vi "CMD_VIDEO.vi"(6 "Gantry in":refnum<class "Gantry.lvclass">, 8 "error in (no error)":errorcluster, 10 "Arguments":string[](array[string]), 11 "gScript Interpreter in":refnum<class "gScript Interpreter.lvclass">) -> (0 "error out":errorcluster, 1 "Pause out":bool, 3 "gScript Interpreter out":refnum<class "gScript Interpreter.lvclass">, 4 "Gantry out":refnum<class "Gantry.lvclass">)   [LabVIEW 2024, in "gScript Interpreter.lvclass"]
uses:
  gScript Interpreter.lvclass
  Shared Components/Gantry Class/Gantry.lvclass
  Shared Components/Vec3d Class/Vec3d.lvclass
  Shared Components/Utils/Type Definitions/Physical Image.ctl
  <vilib>/vision/Image Controls.llb/IMAQ Image.ctl
  Shared Components/FlexWorktable/FlexWorktable.lvclass
  gScript Interpreter.lvclass/gScript Interpreter.ctl
  Shared Components/Vision/Vision.lvlib
panel:
  in  "Snapshot":bool
  in  "Point B Image":refnum<class "Vec3d.lvclass">
  in  "Point A Image":refnum<class "Vec3d.lvclass">
  in  "Point B":refnum<class "Vec3d.lvclass">
  in  "Point A":refnum<class "Vec3d.lvclass">
  in  "Mode Selection":enum32{"Motion", "Measure"}(radio)
  out "Error List":map{string, u64}(c390)
  out "FPS":string
  out "Reference Image":T1(plugin-control)
  in  "Autofocus":bool
  in  "Copy Button":bool
  in  "Pause on Exit":bool
  in  "Light Intensity":i32(slide) scale=0.0..100.0
  in  "Crosshair":bool
  out "Z":dbl format="%.3f"
  out "Y":dbl format="%.3f"
  out "X":dbl format="%.3f"
  in  "Continue":bool
  out "Preview":T1(plugin-control)
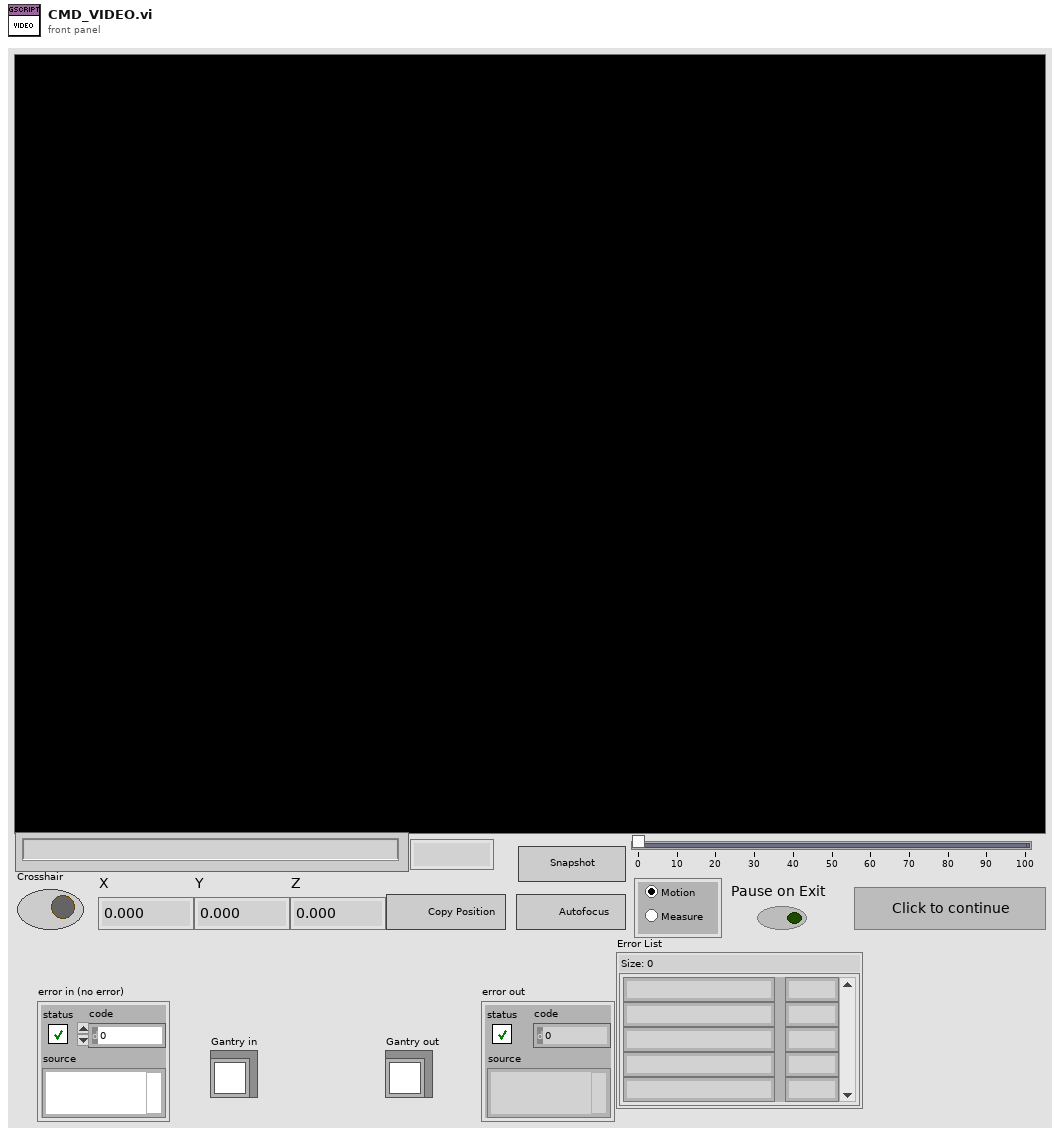
[diagram p1: front panel]
types:
  T1 = typedef "IMAQ Image.ctl" = refnum<image>
  T2 = typedef "Physical Image.ctl" = cluster{"Image Position":refnum<class "Vec3d.lvclass">, "Image Reference":T1, "Field of View":cluster{"x(mm)":dbl, "y(mm)":dbl}}
  T3 = cluster{"Left":i32, "Top":i32, "Right":i32, "Bottom":i32}
  T4 = typedef "FlexWorktable.lvclass/Camera State.ctl" = cluster{"Group":i32, "Open?":bool, "Driver":T5, "serial number":string, "Field of View":cluster{"x-mm":dbl, "y-mm":dbl}, "Rotation":T6, "Vertical Mirror":bool}
  T5 = typedef "Vision.lvlib/camera driver.ctl" = enum16{"none", "wmf", "imaqdx", "peak"}
  T6 = typedef "Camera Rotation.ctl" = enum16{"0", "90", "180", "270"}
  T7 = cluster{"Shift":bool, "Ctrl":bool, "Alt":bool, "Cmd":bool, "Opt":bool}
  T8 = typedef "Vision.lvlib/camera.ctl" = cluster{"camera reference":variant, "driver":T5, "identifier":string}
  T9 = typedef "LVPoint32TypeDef.ctl" = cluster{"Horizontal":i32, "Vertical":i32}
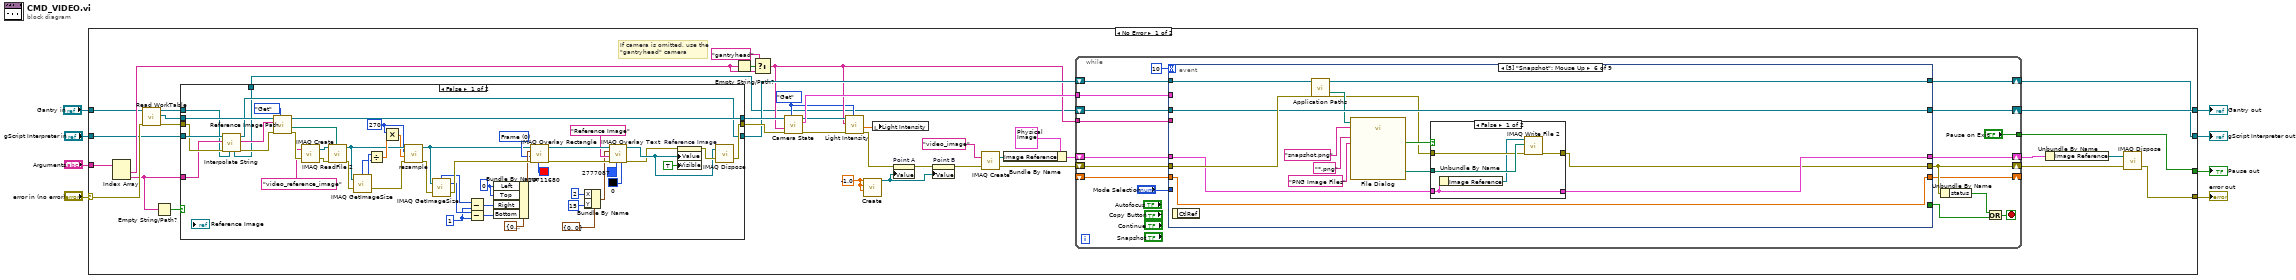
[diagram p0: block diagram]
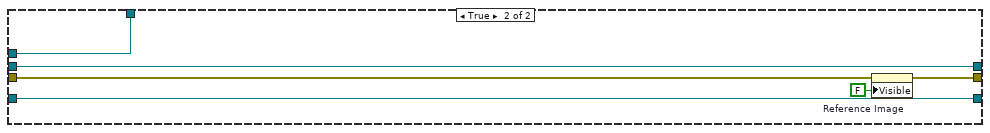
[diagram p2: hidden frame]
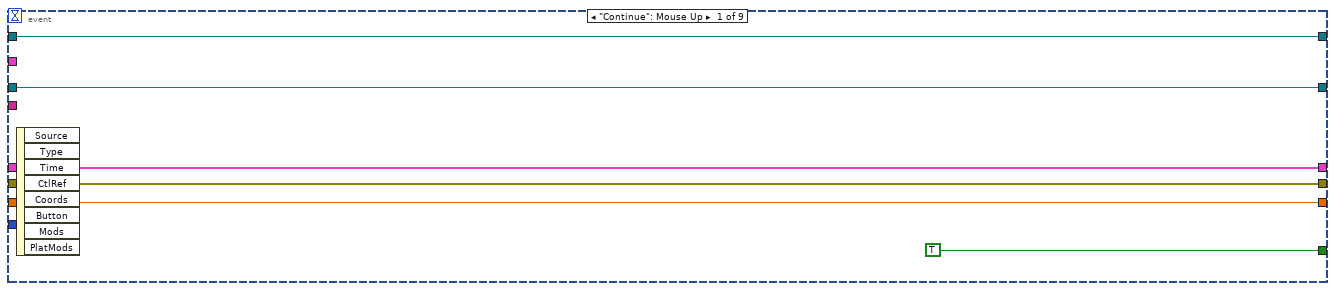
[diagram p3: hidden frame]
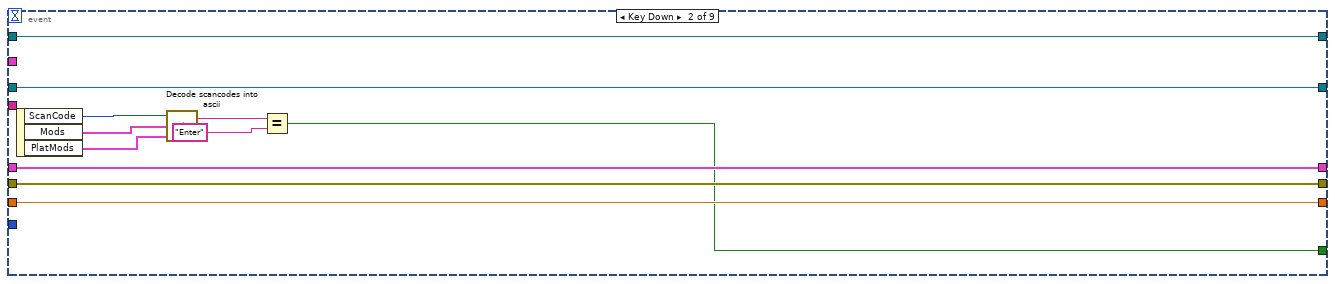
[diagram p4: hidden frame]
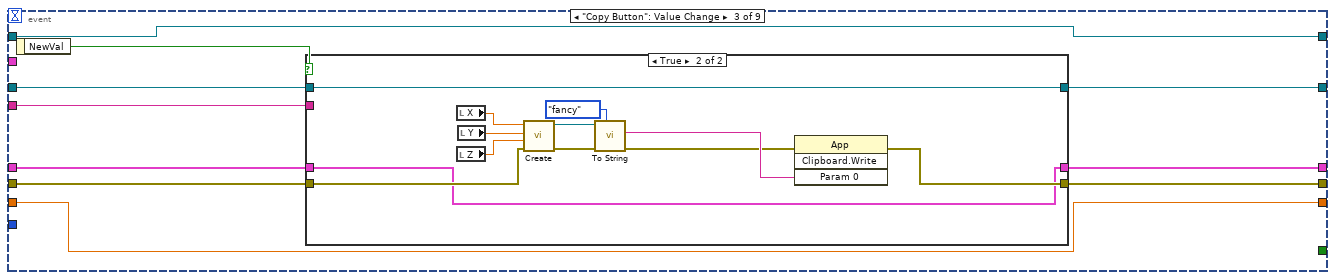
[diagram p5: hidden frame]
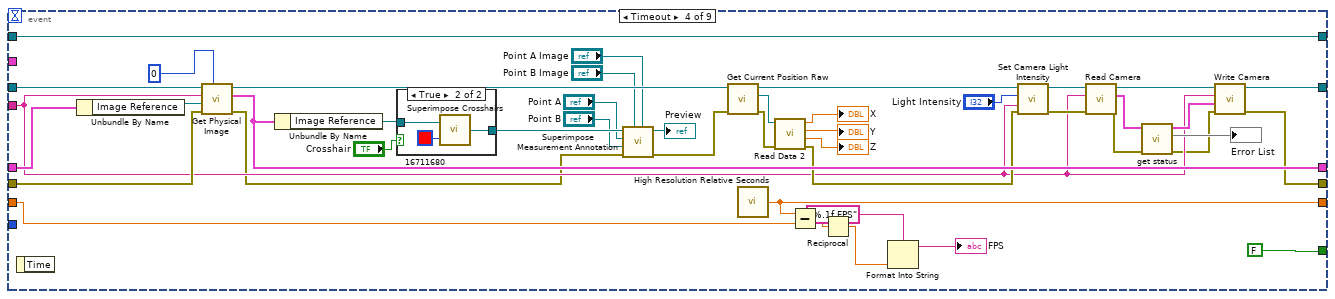
[diagram p7: hidden frame]
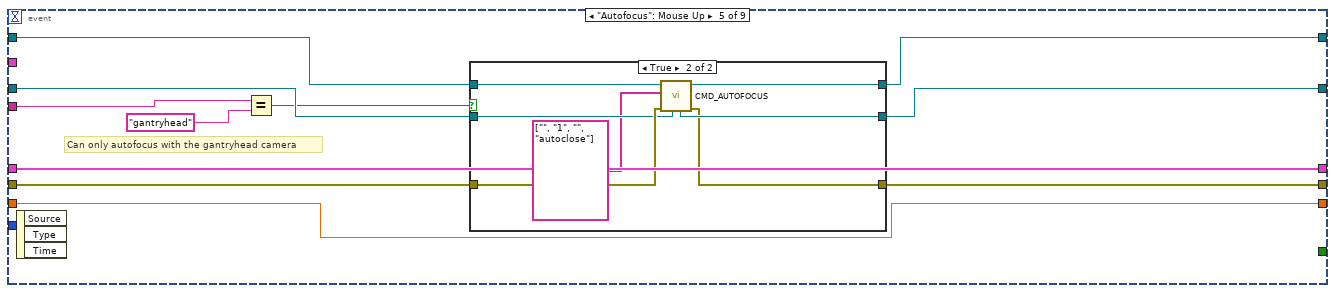
[diagram p9: hidden frame]
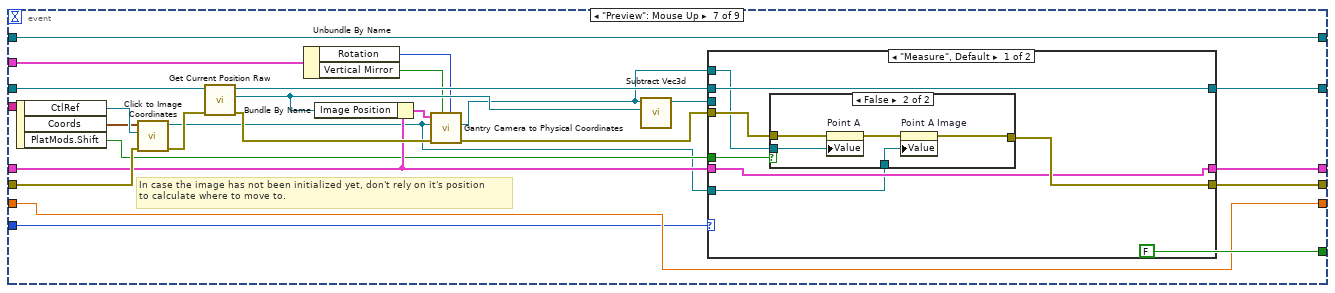
[diagram p12: hidden frame]
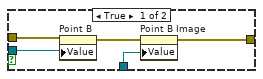
[diagram p13: hidden frame]
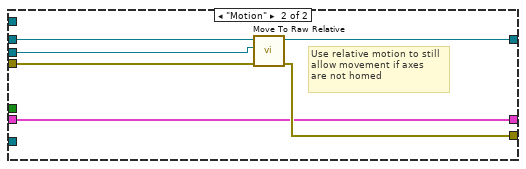
[diagram p14: hidden frame]
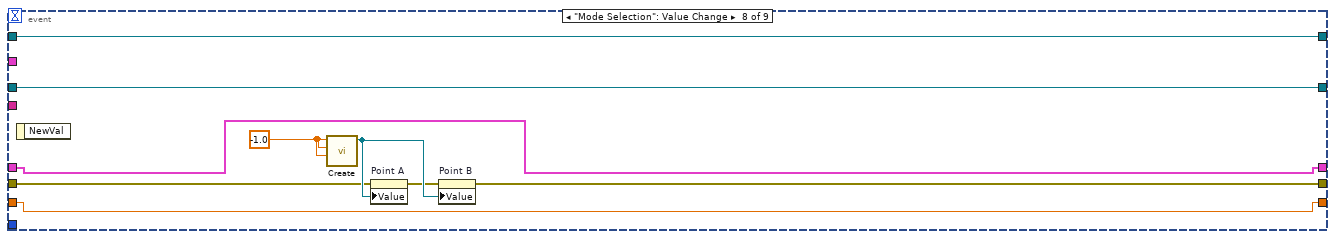
[diagram p15: hidden frame]
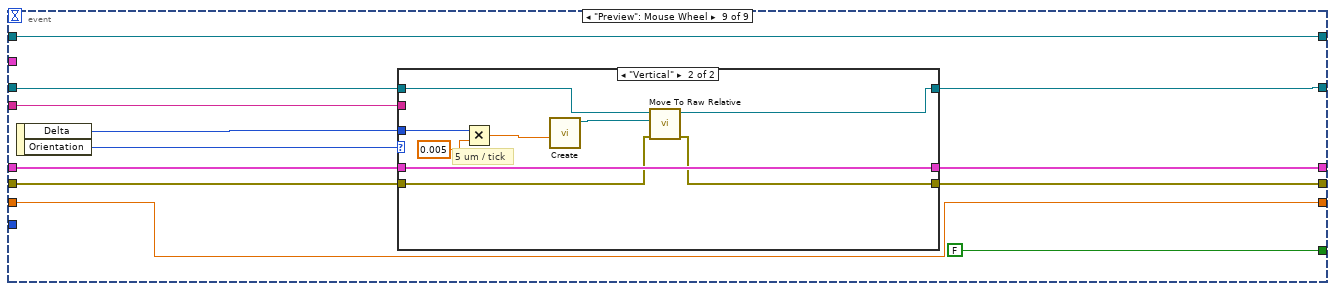
[diagram p16: hidden frame]
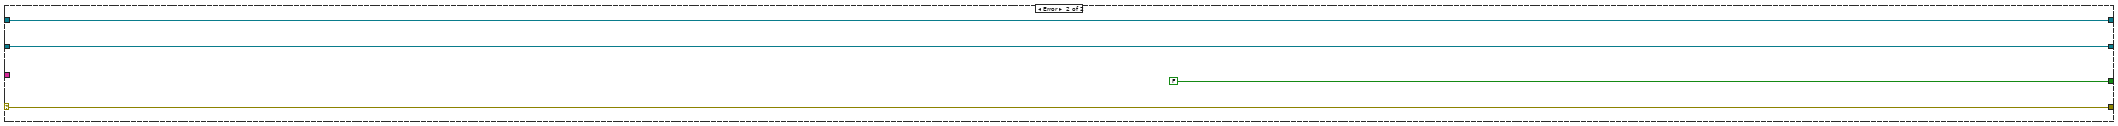
[diagram p18: hidden frame]
diagram:
  n1 = case shown="No Error" "error in (no error)" {
    selector: "error in (no error)" -> [w29 w340]
    tunnel: [w45 w340] -> w7
    tunnel: [w32 w339] -> w5
    tunnel: "gScript Interpreter in" -> [w22 w339]
    tunnel: "Arguments" -> [w47 _]
    tunnel: "Gantry in" -> [w31 w338]
    tunnel: [w46 w338] -> w2
    tunnel: [w33 FALSE ("Pause on Exit")] -> w1
    frame No Error {
      w12 = -1.0 ("X")
      w17 = enum16{"Get", "Set"}."Get" ("Get/Set")
      # "If camera is omitted, use the\n\"gantryhead\" camera"
      n2 = Index Array(array=w47) -> (element #1=w43:string, element #2=w26:string)  [unwired: 2 in]
      n3 = call-dynamic "Read WorkTable.vi"("error in"=w29, "Gantry Class in"=w31) -> ("error out"=w24:errorcluster, "Worktable"=w28:refnum<class "FlexWorktable.lvclass">, "Gantry Class out"=w10:refnum<class "Gantry.lvclass">)  [unwired: 7 in]
      n4 = Empty String/Path?(string/path=w26) -> (empty?=w27:bool)
      n5 = case shown="False" w27 {
        tunnel: w28 -> [w52 w104]
        tunnel: w26 -> [w54 _]
        tunnel: [w92 w104] -> w25
        tunnel: w24 -> [w55 w102]
        tunnel: [w90 w101] -> w23
        tunnel: w22 -> [w56 w100]
        tunnel: [w50 w100] -> w21
        tunnel: w10 -> [w49 w99]
        tunnel: [w48 w99] -> w9
        frame False {
          w58 = 270 ("X Resolution")
          w78 = u32 0 items=["Frame", "Fill", "Highlight"] ("Drawing Mode (Frame)")
          w80 = 1 ("y")
          w85 = 0 ("Left")
          n6 = call-dynamic "Interpolate String.vi"("Gantry in"=w49, "error in (no error)"=w55, "Input String"=w54, "gScript Interpreter in"=w56) -> ("error out"=w51:errorcluster, "Output String"=w53:string, "gScript Interpreter out"=w50:refnum<class "gScript Interpreter.lvclass">, "Gantry out"=w48:refnum<class "Gantry.lvclass">)  [unwired: 4 in]
          n7 = call "Reference Image Path.vi"("Get/Set"=enum16{"Get", "Set"}."Get", "error in (no error)"=w51, "Image ID/Path"=w53, "FlexWorktable in"=w52) -> ("error out"=w95:errorcluster, "Image Path"=w97:path, "FlexWorktable out"=w92:refnum<class "FlexWorktable.lvclass">)  [unwired: 5 in]
          n8 = call "IMAQ Create"("Image Name"="video_reference_image", "error in (no error)"=w95) -> ("New Image"=w96:T1, "error out"=w94:errorcluster)  [unwired: 3 in]
          n9 = call "IMAQ ReadFile 2"("File Path"=w97, "error in (no error)"=w94, "Image"=w96) -> ("error out"=w66:errorcluster, "Image Out"=w60:T1)  [unwired: 4 in, 3 out]
          n10 = call "IMAQ GetImageSize"("Image"=w60, "error in (no error)"=w66) -> ("Y Resolution"=w65:i32, "X Resolution"=w64:i32, "error out"=w61:errorcluster)  [unwired: 2 in]
          n11 = Divide(x=w65, y=w64) -> (x/y=w63:dbl)
          n12 = Multiply(x=w58, y=w63) -> (x*y=w57:dbl)
          n13 = call "resample.vi"("error in (no error)"=w61, "Height"=w57, "Width"=w58, "Image in"=w60) -> ("error out"=w62:errorcluster, "Image out"=w59:T1)  [unwired: 6 in]
          n14 = call "IMAQ GetImageSize"("Image"=w59, "error in (no error)"=w62) -> ("Y Resolution"=w81:i32, "X Resolution"=w82:i32, "error out"=w87:errorcluster)  [unwired: 2 in]
          n15 = Subtract(x=w82, y=w80) -> (x-y=w83:i32)
          n16 = Subtract(x=w81, y=w80) -> (x-y=w79:i32)
          n17 = Bundle By Name(cluster=T3 {"Left"=0, "Top"=0, "Right"=0, "Bottom"=0} ("Rectangle"), "Left"=w85, "Top"=w85, "Right"=w83, "Bottom"=w79) -> (w84:T3)
          n18 = call "IMAQ Overlay Rectangle"("Color"=u32 16711680, "error in (no error)"=w87, "Drawing Mode (Frame)"=w78, "Rectangle"=w84, "Image"=w59) -> ("error out"=w77:errorcluster, "Image Out"=w76:T1)  [unwired: 5 in]
          n19 = Bundle By Name(cluster=cluster{"X":i32, "Y":i32} {"X"=0, "Y"=0} ("Origin"), "X"=2, "Y"=15) -> (w69:cluster{"X":i32, "Y":i32})
          n20 = call "IMAQ Overlay Text"("BG Color (Transparent)"=u32 0, "Text Color (black)"=u32 2777087, "error in (no error)"=w77, "String"="Reference Image", "Origin"=w69, "Image"=w76) -> ("error out"=w74:errorcluster, "Image Out"=w75:T1)  [unwired: 4 in]
          n21 = property on="Reference Image" class="ImageControl"(error in=w74, "Value"=w75, "Visible"=TRUE) -> (error out=w91:errorcluster)  [unwired: 1 in, 1 out]
          n22 = call "IMAQ Dispose"("Image"=w75, "error in (no error)"=w91) -> ("error out"=w90:errorcluster)  [unwired: 4 in]
        }
        frame True {
          n23 = property on="Reference Image" class="ImageControl"(error in=w102, "Visible"=FALSE) -> (error out=w101:errorcluster)  [unwired: 1 in, 1 out]
        }
      }
      n24 = Empty String/Path?(string/path=w43) -> (empty?=w44:bool)
      n25 = Select(t="gantryhead", s=w44, f=w43) -> (s? t:f=w18:string)
      n26 = call-dynamic "Camera State.vi"("Get/Set"=w17, "error in (no error)"=w23, "Camera Name"=w18, "FlexWorktable in"=w25) -> ("error out"=w20:errorcluster, "State"=w30:T4, "FlexWorktable out"=w19:refnum<class "FlexWorktable.lvclass">)  [unwired: 5 in]
      n27 = call "Light Intensity.vi"("Get/Set"=w17, "error in (no error)"=w20, "Light Name"=w18, "FlexWorktable in"=w19) -> ("error out"=w15:errorcluster, "Intensity out"=w16:dbl)  [unwired: 5 in, 1 out]
      n28 = call "Create.vi"("Z"=w12, "Y"=w12, "X"=w12) -> ("Vec3d Class out"=w11:refnum<class "Vec3d.lvclass">)  [unwired: 7 in, 1 out]
      n29 = local write "Light Intensity"(w16) -> ()
      n30 = property on="Point A" class="LVClassControl (strict)"(error in=w15, "Value"=w11) -> (error out=w14:errorcluster)  [unwired: 1 in, 1 out]
      n31 = property on="Point B" class="LVClassControl (strict)"(error in=w14, "Value"=w11) -> (error out=w13:errorcluster)  [unwired: 1 in, 1 out]
      n32 = call "IMAQ Create"("Image Name"="video_image", "error in (no error)"=w13) -> ("New Image"=w38:T1, "error out"=w40:errorcluster)  [unwired: 3 in]
      n33 = Bundle By Name(cluster=T2 {"Image Position"=refnum, "Image Reference"=refnum, "Field of View"={"x(mm)"=0.0, "y(mm)"=0.0}} ("Physical Image"), "Image Reference"=w38) -> (w37:T2)
      n34 = while {
        shift-right: [w117] -> w46
        shift-left: w9 -> [w118]
        tunnel: w18 -> [w119]
        shift-right: [w116] -> w36
        shift-left: w37 -> [w120]
        shift-right: [w115] -> w34
        shift-left: w40 -> [w121]
        tunnel: ["Pause on Exit"] -> w33
        shift-right: [w110] -> w32
        shift-left: w21 -> [w111]
        tunnel: w30 -> [w109]
        shift-right: [w108] -> _
        shift-left: _ -> [w107]
        stop <- w112 stop-if-true
        n35 = event shown="[5] \"Snapshot\": Mouse Up" {
          selector: _ -> [_ _ _ _ _ _ _ _ _]
          dyn-events: _ -> [_ _ _ _ _ _ _ _ _]
          timeout: 10 -> [_ _ _ _ _ _ _ _ _]
          tunnel: w121 -> [w125 w137 w145 w199 w222 w246 w278 w307 w321]
          tunnel: w120 -> [w126 w138 w146 w198 w217 w243 w260 w305 w323]
          tunnel: w119 -> [_ _ w147 w176 w216 _ _ _ w316]
          tunnel: [w127 w139 w144 w173 w220 w238 w270 w308 w317] -> w117
          tunnel: w118 -> [w127 w139 w148 w200 w221 w238 w276 w308 w318]
          tunnel: [w126 w138 w143 w196 w217 w239 w259 w305 w322] -> w116
          tunnel: [w125 w137 w142 w174 w218 w237 w266 w306 w320] -> w115
          tunnel: [TRUE w129 _ FALSE _ _ FALSE _ FALSE] -> w113
          tunnel: w111 -> [w124 w136 w141 w190 w223 w248 w275 w312 w314]
          tunnel: [w124 w136 w141 w190 w219 w247 w275 w312 w314] -> w110
          tunnel: w109 -> [_ _ _ _ _ _ w265 _ _]
          tunnel: [w123 w135 w140 w189 w213 w236 w262 w304 w313] -> w108
          tunnel: w107 -> [w123 w135 w140 w188 w213 w236 w262 w304 w313]
          tunnel: "Mode Selection" -> [_ _ _ _ _ _ w261 _ _]
          event "Continue": Mouse Up {
            n36 = event-data() -> ()  [unwired: 1 in, 8 out]
          }
          event Key Down {
            n37 = event-data() -> ("ScanCode"=w134:i16, "Mods"=w133:cluster{"Num Pad":bool, "Menu Key":bool}, "PlatMods"=w132:T7)  [unwired: 1 in]
            n38 = call "Decode scancodes into ascii.vi"("PlatMods"=w132, "Mods"=w133, "ScanCode"=w134) -> ("String"=w131:string)  [unwired: 1 out]
            n39 = Equal?(x=w131, y="Enter") -> (x = y?=w129:bool)
          }
          event "Copy Button": Value Change {
            n40 = event-data() -> ("NewVal"=w149:bool)  [unwired: 1 in]
            n41 = case shown="True" w149 {
              tunnel: w148 -> [w152 w164]
              tunnel: w147 -> [_ _]
              tunnel: w146 -> [w151 w153]
              tunnel: w145 -> [w150 w158]
              tunnel: [w152 w164] -> w144
              tunnel: [w151 w153] -> w143
              tunnel: [w150 w154] -> w142
              frame False {
              }
              frame True {
                n42 = local read "X"() -> (w163:dbl)
                n43 = local read "Z"() -> (w161:dbl)
                n44 = local read "Y"() -> (w162:dbl)
                n45 = call "Create.vi"("error in"=w158, "Z"=w161, "Y"=w162, "X"=w163) -> ("error out"=w157:errorcluster, "Vec3d Class out"=w160:refnum<class "Vec3d.lvclass">)  [unwired: 6 in]
                n46 = call "To String.vi"("Formatting"=enum16{"plain", "fancy"}."fancy", "error in"=w157, "Vec3d in"=w160) -> ("error out"=w155:errorcluster, "Vec3d String"=w156:string)  [unwired: 6 in, 1 out]
                n47 = invoke class="App" method="Clipboard.Write"(error in=w155, "Param 0"=w156) -> (error out=w154:errorcluster)  [unwired: 2 in, 3 out]
              }
            }
          }
          event Timeout {
            n48 = event-data() -> ()  [unwired: 1 in, 1 out]
            n49 = Unbundle By Name(w198) -> ("Image Reference"=w197:T1)
            n50 = call-dynamic "Get Physical Image.vi"("Delay(milliseconds)"=0, "error in"=w199, "Image In"=w197, "Camera Name"=w176, "Gantry in"=w200) -> ("error out"=w171:errorcluster, "Physical Image"=w196:T2, "Gantry out"=w201:refnum<class "Gantry.lvclass">)  [unwired: 4 in]
            n51 = Unbundle By Name(w196) -> ("Image Reference"=w195:T1)
            n52 = case shown="True" "Crosshair" {
              tunnel: w195 -> [w209 w210]
              tunnel: [w209 w211] -> w172
              frame False {
              }
              frame True {
                n53 = call "Superimpose Crosshairs.vi"("Grid Line Color"=u32 16711680, "Refnum in"=w210) -> ("Refnum out"=w211:T1)  [unwired: 1 in]
              }
            }
            n54 = call "Superimpose Measurement Annotation.vi"("Point A Image"="Point A Image", "Point B Image"="Point B Image", "error in"=w171, "Point B"="Point B", "Point A"="Point A", "Image In"=w172) -> ("error out"=w170:errorcluster, "Image Out"=→"Preview":T1)  [unwired: 4 in]
            n55 = call-dynamic "Get Current Position Raw.vi"("error in"=w170, "Gantry in"=w201) -> ("error out"=w206:errorcluster, "Vec3d Class out"=w207:refnum<class "Vec3d.lvclass">, "Gantry out"=w193:refnum<class "Gantry.lvclass">)  [unwired: 7 in]
            n56 = call <vilib>:"High Resolution Relative Seconds.vi"() -> ("relative seconds"=w189:dbl)
            n57 = call-dynamic "Read Data 2.vi"("error in"=w206, "Vec3d in"=w207) -> ("error out"=w191:errorcluster, "Z"=→"Z":dbl, "Y"=→"Y":dbl, "X"=→"X":dbl)  [unwired: 6 in]
            n58 = Subtract(x=w189, y=w188) -> (x-y=w187:dbl)
            n59 = Reciprocal(x=w187) -> (1/x=w186:dbl)
            n60 = Format Into String(format string="%.1f FPS", w186) -> (resulting string=→"FPS":string)  [unwired: 2 in, 1 out]
            n61 = call-dynamic "Set Camera Light Intensity.vi"("error in (no error)"=w191, "camera name"=w176, "Intensity"="Light Intensity", "Gantry Class in"=w193) -> ("error out"=w182:errorcluster, "Gantry Class out"=w183:refnum<class "Gantry.lvclass">)  [unwired: 6 in]
            n62 = call-dynamic "Read Camera.vi"("error in (no error)"=w182, "Camera Name"=w176, "Gantry Class in"=w183) -> ("error out"=w179:errorcluster, "Camera"=w181:T8, "Gantry Class out"=w178:refnum<class "Gantry.lvclass">)  [unwired: 6 in]
            n63 = call "get status.vi"("error in (no error)"=w179, "Camera"=w181) -> ("error out"=w175:errorcluster, "Error List"=→"Error List":map{string, u64}, "Camera out"=w177:T8)  [unwired: 7 in]
            n64 = call-dynamic "Write Camera.vi"("error in (no error)"=w175, "Camera"=w177, "Camera Name"=w176, "Gantry Class in"=w178) -> ("error out"=w174:errorcluster, "Gantry Class out"=w173:refnum<class "Gantry.lvclass">)  [unwired: 6 in]
          }
          event "Autofocus": Mouse Up {
            # "Can only autofocus with the gantryhead camera"
            n65 = event-data() -> ()  [unwired: 1 in, 3 out]
            n66 = Equal?(x=w216, y="gantryhead") -> (x = y?=w214:bool)
            n67 = case shown="True" w214 {
              tunnel: w223 -> [w226 w233]
              tunnel: w222 -> [w224 w232]
              tunnel: w221 -> [w225 w231]
              tunnel: [w225 w230] -> w220
              tunnel: [w226 w229] -> w219
              tunnel: [w224 w228] -> w218
              frame False {
              }
              frame True {
                n68 = call-dynamic "CMD_AUTOFOCUS.vi"("Gantry in"=w231, "error in (no error)"=w232, "Arguments"=string[] ["", "1", "", "autoclose"], "gScript Interpreter in"=w233) -> ("error out"=w228:errorcluster, "gScript Interpreter out"=w229:refnum<class "gScript Interpreter.lvclass">, "Gantry out"=w230:refnum<class "Gantry.lvclass">)  [unwired: 5 in]
              }
            }
          }
          event "Snapshot": Mouse Up {
            n69 = event-data() -> ()  [unwired: 1 in, 1 out]
            n70 = call "Application Paths.vi"("gScript Interpreter in"=w248, "error in (no error)"=w246) -> ("gScript Interpreter out"=w247:refnum<class "gScript Interpreter.lvclass">, "Logs Path"=w235:path, "error out"=w234:errorcluster)  [unwired: 12 in, 3 out]
            n71 = call "File Dialog"("start path"=w235, "default name"="snapshot.png", "pattern (all files)"="*.png" ("pattern label"), "pattern label"="PNG Image Files") -> ("selected path"=w244:path, "cancelled"=w245:bool)  [unwired: 8 in, 2 out]
            n72 = case shown="False" w245 {
              tunnel: w244 -> [w253 _]
              tunnel: w234 -> [w252 w254]
              tunnel: w243 -> [w250 w255]
              tunnel: [w250 w255] -> w239
              tunnel: [w249 w254] -> w237
              frame False {
                n73 = Unbundle By Name(w250) -> ("Image Reference"=w251:T1)
                n74 = call-poly "IMAQ Write File 2"("error in (no error)"=w252, "File Path"=w253, "Image"=w251) -> ("error out"=w249:errorcluster)  [unwired: 7 in, 1 out]
              }
              frame True {
              }
            }
          }
          event "Preview": Mouse Up {
            # "In case the image has not been initialized yet, don't rely on it's position\nto calculate where to move to."
            n75 = event-data() -> ("CtlRef"=w280:refnum<vi>, "Coords"=w279:T9, "PlatMods.Shift"=w258:bool)  [unwired: 1 in]
            n76 = call "Click to Image Coordinates.vi"("error in"=w278, "Display Reference"=w280, "Coords"=w279) -> ("error out"=w273:errorcluster, "Image Coordinates"=w257:refnum<class "Vec3d.lvclass">)  [unwired: 7 in]
            n77 = call-dynamic "Get Current Position Raw.vi"("error in"=w273, "Gantry in"=w276) -> ("error out"=w272:errorcluster, "Vec3d Class out"=w268:refnum<class "Vec3d.lvclass">, "Gantry out"=w271:refnum<class "Gantry.lvclass">)  [unwired: 7 in]
            n78 = Unbundle By Name(w265) -> ("Rotation"=w264:T6, "Vertical Mirror"=w263:bool)
            n79 = Bundle By Name(cluster=w260, "Image Position"=w268) -> (w274:T2)
            n80 = call "Gantry Camera to Physical Coordinates.vi"("Rotation"=w264, "Vertical Mirror"=w263, "error in"=w272, "Image Coordinate"=w257, "Physical Image"=w274) -> ("error out"=w267:errorcluster, "Global Coordinate"=w256:refnum<class "Vec3d.lvclass">)  [unwired: 4 in, 1 out]
            n81 = call "Subtract Vec3d.vi"("Vec3d in 2"=w268, "Vec3d in 1"=w256) -> ("Vec3d Class out"=w269:refnum<class "Vec3d.lvclass">)  [unwired: 8 in, 1 out]
            n82 = case shown="\"Measure\", Default" w261 {
              tunnel: w271 -> [w287 w303]
              tunnel: [w287 w302] -> w270
              tunnel: w269 -> [_ w301]
              tunnel: w267 -> [w286 w300]
              tunnel: [w284 w299] -> w266
              tunnel: w260 -> [w283 w298]
              tunnel: [w283 w298] -> w259
              tunnel: w258 -> [w285 _]
              tunnel: w257 -> [w282 _]
              tunnel: w256 -> [w281 _]
              frame "Measure", Default {
                n83 = case shown="False" w285 {
                  tunnel: w281 -> [w291 w297]
                  tunnel: w286 -> [w292 w296]
                  tunnel: [w289 w294] -> w284
                  tunnel: w282 -> [w288 w293]
                  frame True {
                    n84 = property on="Point B" class="LVClassControl (strict)"(error in=w292, "Value"=w291) -> (error out=w290:errorcluster)  [unwired: 1 in, 1 out]
                    n85 = property on="Point B Image" class="LVClassControl (strict)"(error in=w290, "Value"=w288) -> (error out=w289:errorcluster)  [unwired: 1 in, 1 out]
                  }
                  frame False {
                    n86 = property on="Point A" class="LVClassControl (strict)"(error in=w296, "Value"=w297) -> (error out=w295:errorcluster)  [unwired: 1 in, 1 out]
                    n87 = property on="Point A Image" class="LVClassControl (strict)"(error in=w295, "Value"=w293) -> (error out=w294:errorcluster)  [unwired: 1 in, 1 out]
                  }
                }
              }
              frame "Motion" {
                # "Use relative motion to still\nallow movement if axes\nare not homed"
                n88 = call-dynamic "Move To Raw Relative.vi"("error in"=w300, "Delta"=w301, "Gantry in"=w303) -> ("error out"=w299:errorcluster, "Gantry out"=w302:refnum<class "Gantry.lvclass">)  [unwired: 7 in]
              }
            }
          }
          event "Mode Selection": Value Change {
            w309 = -1.0 ("X")
            n89 = event-data() -> ()  [unwired: 1 in, 1 out]
            n90 = call "Create.vi"("Z"=w309, "Y"=w309, "X"=w309) -> ("Vec3d Class out"=w311:refnum<class "Vec3d.lvclass">)  [unwired: 7 in, 1 out]
            n91 = property on="Point A" class="LVClassControl (strict)"(error in=w307, "Value"=w311) -> (error out=w310:errorcluster)  [unwired: 1 in, 1 out]
            n92 = property on="Point B" class="LVClassControl (strict)"(error in=w310, "Value"=w311) -> (error out=w306:errorcluster)  [unwired: 1 in, 1 out]
          }
          event "Preview": Mouse Wheel {
            n93 = event-data() -> ("Delta"=w324:i32, "Orientation"=w315:enum16{"Horizontal", "Vertical"})  [unwired: 1 in]
            n94 = case shown="\"Vertical\"" w315 {
              tunnel: w324 -> [_ w330]
              tunnel: w323 -> [w326 w336]
              tunnel: [w326 w336] -> w322
              tunnel: w321 -> [w327 w333]
              tunnel: [w327 w332] -> w320
              tunnel: w318 -> [w325 w335]
              tunnel: [w325 w334] -> w317
              tunnel: w316 -> [_ _]
              frame "Horizontal", Default {
              }
              frame "Vertical" {
                # "5 um / tick"
                n95 = Multiply(x=w330, y=0.005) -> (x*y=w328:dbl)
                n96 = call "Create.vi"("Z"=w328) -> ("Vec3d Class out"=w331:refnum<class "Vec3d.lvclass">)  [unwired: 9 in, 1 out]
                n97 = call-dynamic "Move To Raw Relative.vi"("error in"=w333, "Delta"=w331, "Gantry in"=w335) -> ("error out"=w332:errorcluster, "Gantry out"=w334:refnum<class "Gantry.lvclass">)  [unwired: 7 in]
              }
            }
          }
        }
        n98 = Unbundle By Name(w115) -> ("status"=w114:bool)
        n99 = Or(x=w114, y=w113) -> (x .or. y?=w112:bool)
      }
      n100 = Unbundle By Name(w36) -> ("Image Reference"=w35:T1)
      n101 = call "IMAQ Dispose"("Image"=w35, "error in (no error)"=w34) -> ("error out"=w45:errorcluster)  [unwired: 4 in]
    }
    frame Error {
    }
  }
  "error out" <- w7
  "gScript Interpreter out" <- w5
  "Gantry out" <- w2
  "Pause out" <- w1
